vi "Path log testing.vi"() -> ()   [LabVIEW 2015]
panel:
  out "error out":errorcluster
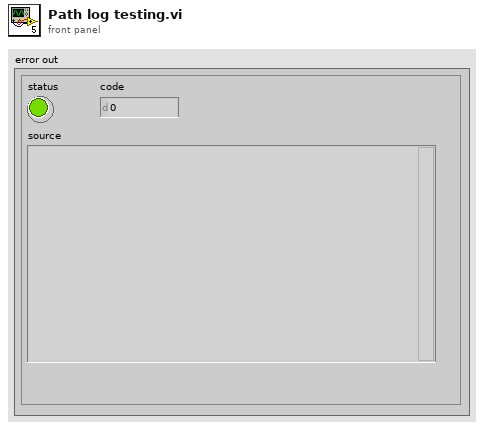
[diagram p1: front panel]
types:
  T1 = enum16{"open", "replace", "create", "open or create", "replace or create", "replace or create with confirmation"}
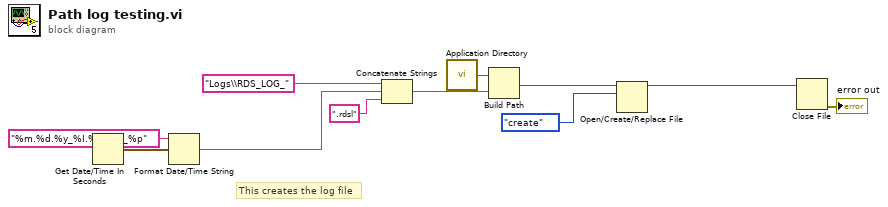
[diagram p0: block diagram]
diagram:
  # "This creates the log file"
  n1 = Get Date/Time In Seconds() -> (seconds since 1Jan1904=w9:timestamp)
  n2 = Format Date/Time String(time format string (%c)="%m.%d.%y_%I.%M.%S_%p", seconds (now)=w9) -> (date/time string=w8:string)  [unwired: 1 in]
  n3 = Concatenate Strings("Logs\\RDS_LOG_" ("name or relative path"), w8, ".rdsl" ("string")) -> (w5:string)
  n4 = call <vilib>:"Application Directory.vi"() -> ("Application Directory"=w10:path)
  n5 = Build Path(base path=w10, name or relative path=w5) -> (appended path=w4:path)
  n6 = Open/Create/Replace File(file path (use dialog)=w4, operation (0:open)=T1."create") -> (refnum out=w1:refnum<file>)  [unwired: 4 in, 2 out]
  n7 = Close File(refnum=w1) -> (error out=→"error out":errorcluster)  [unwired: 1 in, 1 out]
